vi "CASO.vi"() -> ()   [LabVIEW 2019]
uses:
  <vilib>/ActorFramework/Stop Msg/Stop Msg.lvclass
panel:
  in  "COMPRAR MERCANCÍA":bool
  in  "10 PESOS MEXICANOS":bool
  in  "5 PESOS MEXICANOS":bool
  in  "2 PESOS MEXICANOS":bool
  in  "1 PESO MEXICANO":bool
  in  "SOLICITAR MERCANCIA":bool
  out "PRECIO":dbl
  out "CANTIDAD":dbl
  out "PRODUCTO":string
  out "MONEDA":string
  in  "MERCANCÍA":i32(listbox)
  out "CRÉDITO":dbl
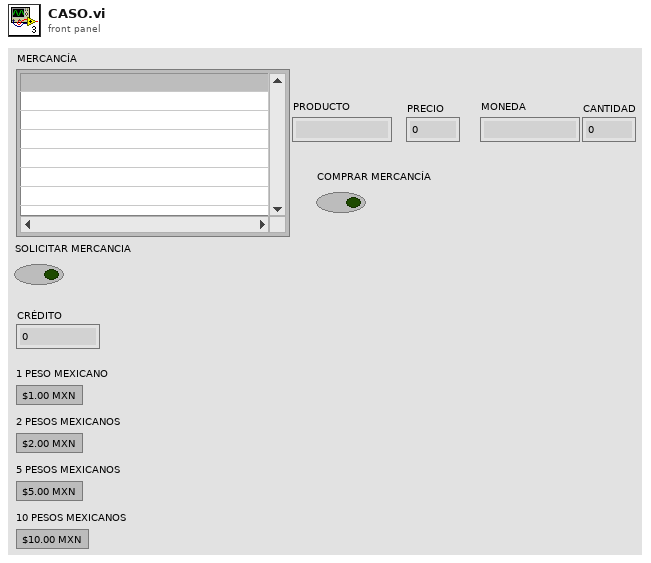
[diagram p1: front panel]
types:
  T1 = cluster{"CANTIDAD":dbl, "MONEDA":string, "PRECIO ":dbl, "PRODUCTO":string}
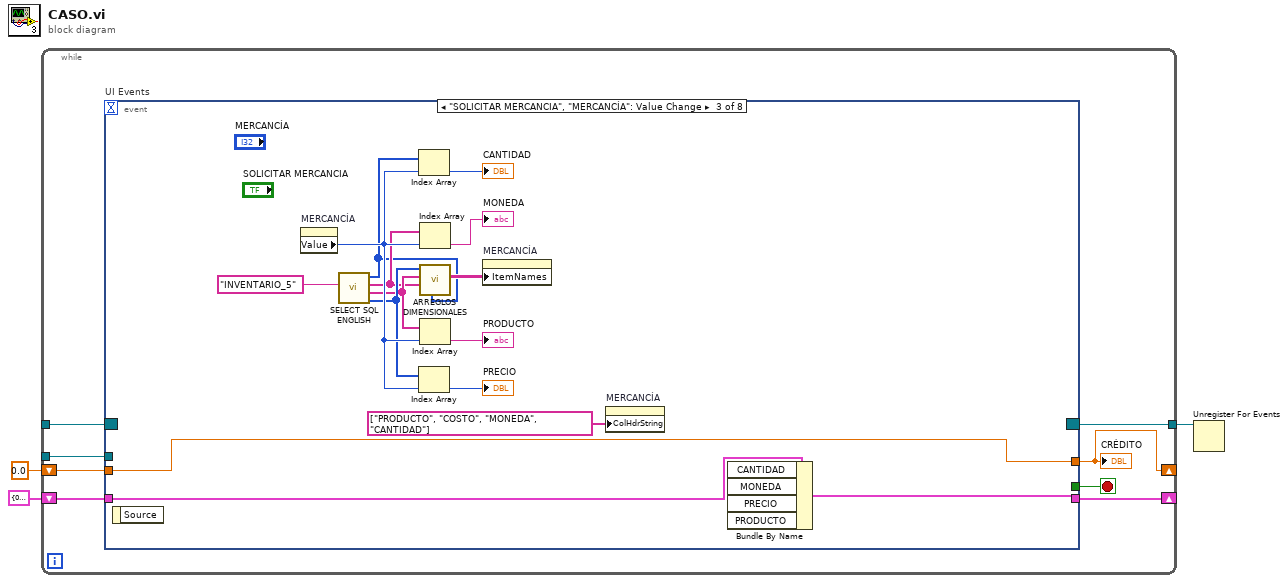
[diagram p0: block diagram]
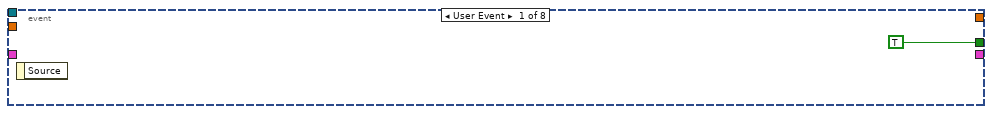
[diagram p2: hidden frame]
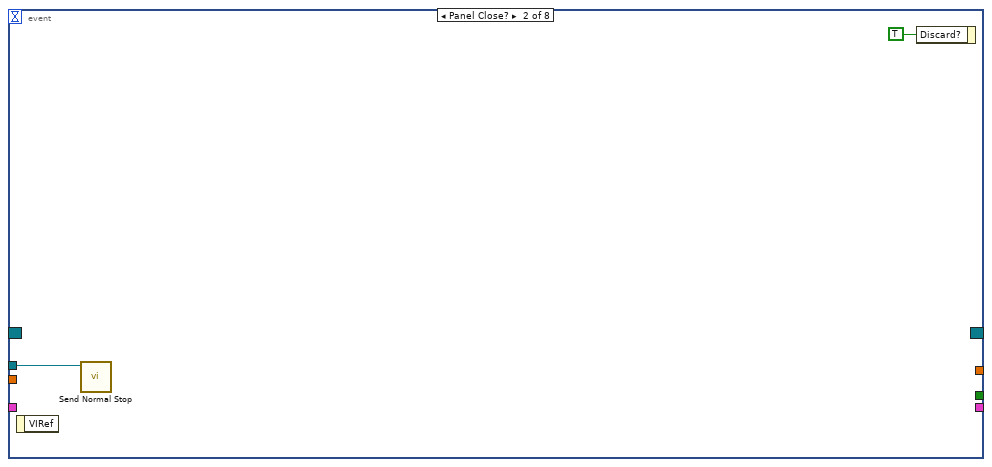
[diagram p3: hidden frame]
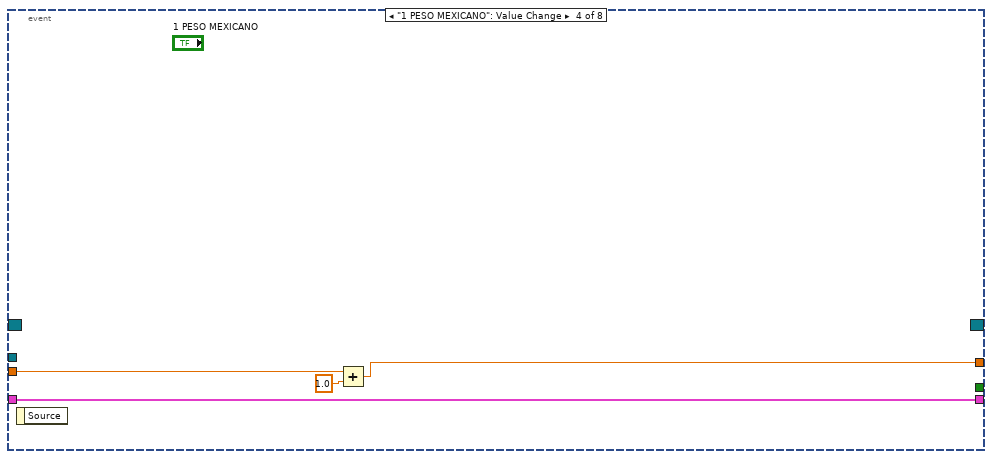
[diagram p4: hidden frame]
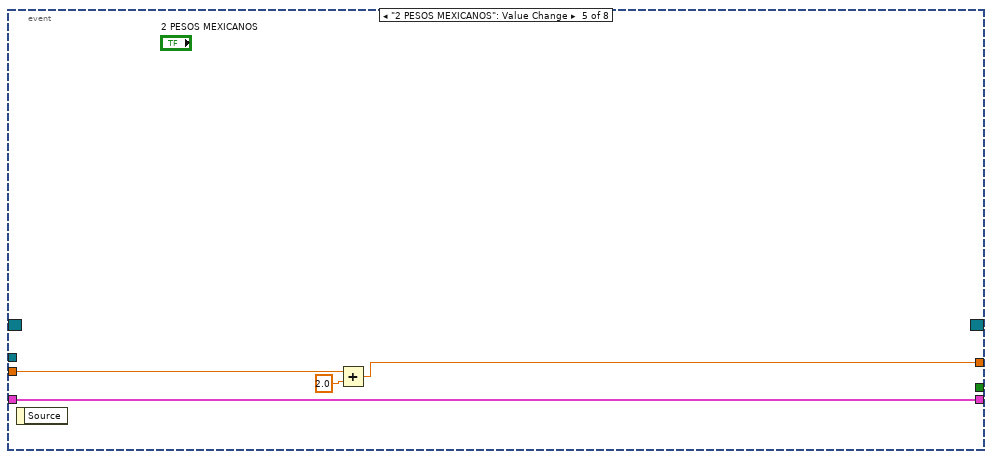
[diagram p5: hidden frame]
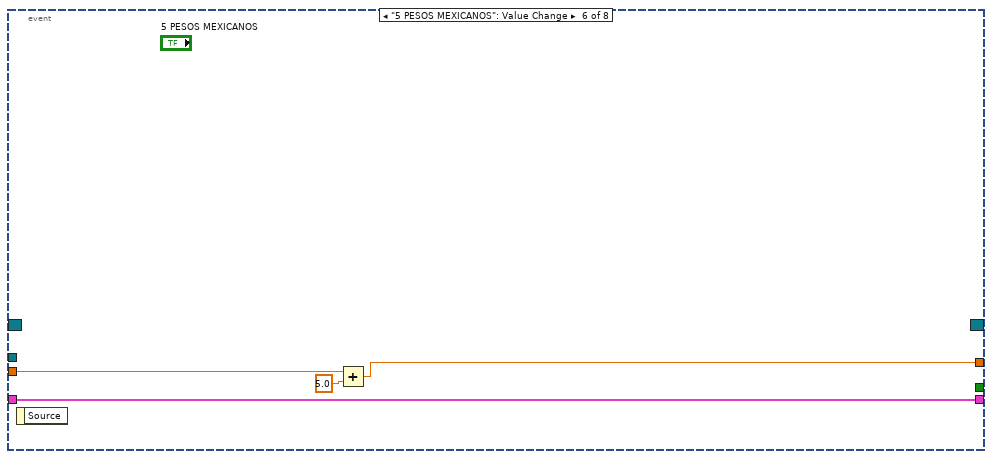
[diagram p6: hidden frame]
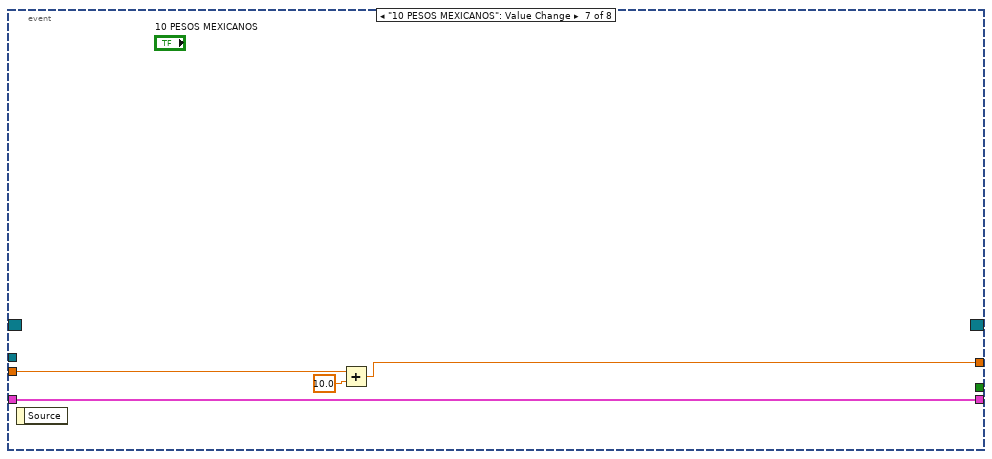
[diagram p7: hidden frame]
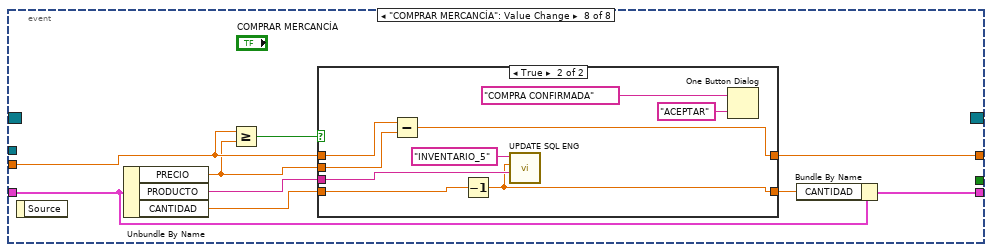
[diagram p8: hidden frame]
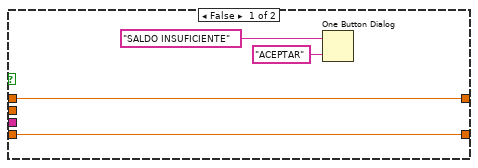
[diagram p9: hidden frame]
diagram:
  n1 = while {
    tunnel: [w12] -> w2
    tunnel: [w10] -> w1
    tunnel: _ -> [w9]
    shift-right: [w7] -> _
    shift-left: T1 {"CANTIDAD"=0.0, "MONEDA"="", "PRECIO "=0.0, "PRODUCTO"=""} -> [w8]
    shift-right: [w5] -> _
    shift-left: 0.0 -> [w6]
    stop <- w11 stop-if-true
    n2 = event "UI Events" shown="[2] \"SOLICITAR MERCANCIA\", \"MERCANCÍA\": Value Change" {
      selector: w12 -> [_ _ _ _ _ _ _ _]
      dyn-events: [_ _ _ _ _ _ _ _] -> w10
      timeout: _ -> [_ _ _ _ _ _ _ _]
      tunnel: [TRUE _ _ _ _ _ _ _] -> w11
      tunnel: w9 -> [_ w14 _ _ _ _ _ _]
      tunnel: w8 -> [_ _ w28 w34 w38 w42 w46 w55]
      tunnel: [_ _ w27 w34 w38 w42 w46 w51] -> w7
      tunnel: [_ _ w25 w31 w35 w39 w43 w47] -> w5
      tunnel: w6 -> [_ _ w25 w33 w37 w41 w45 w49]
      event User Event {
        n3 = event-data() -> ()  [unwired: 1 in, 1 out]
      }
      event Panel Close? {
        n4 = event-data() -> ()  [unwired: 1 in, 1 out]
        n5 = call <vilib>:"Send Normal Stop.vi"("Message Enqueuer"=w14) -> ()  [unwired: 10 in, 1 out]
        n6 = event-data("Discard?"=TRUE) -> ()  [unwired: 1 in, 1 out]
      }
      event "SOLICITAR MERCANCIA", "MERCANCÍA": Value Change {
        n7 = event-data() -> ()  [unwired: 1 in, 1 out]
        n8 = property on="MERCANCÍA" class="MCListbox (strict)"() -> ("Value"=w26:i32)  [unwired: 2 in, 2 out]
        n9 = call "SELECT SQL ENGLISH.vi"("INVENTARIO"="INVENTARIO_5") -> ("COSTO"=w19:i64[], "PRODUCTO"=w18:string[], "MONEDA"=w17:string[], "CANTIDAD"=w16:i64[])  [unwired: 7 in]
        n10 = Index Array(array=w16, index=w26) -> (element=→"CANTIDAD":i64)
        n11 = Index Array(array=w19, index=w26) -> (element=→"PRECIO":i64)
        n12 = Index Array(array=w17, index=w26) -> (element=→"MONEDA":string)
        n13 = call "ARREGLOS DIMENSIONALES.vi"("CANTIDAD"=w16, "MONEDA"=w17, "PRODUCTO"=w18, "COSTO"=w19) -> ("Array"=w29:string[][])  [unwired: 7 in]
        n14 = Index Array(array=w18, index=w26) -> (element=→"PRODUCTO":string)
        n15 = property on="MERCANCÍA" class="MCListbox (strict)"("ItemNames"=w29) -> ()  [unwired: 2 in, 2 out]
        n16 = property on="MERCANCÍA" class="MCListbox (strict)"("ColHdrString"=string[] ["PRODUCTO", "COSTO", "MONEDA", "CANTIDAD"] ("Column Header Strings[]")) -> ()  [unwired: 2 in, 2 out]
        n17 = Bundle By Name(cluster=w28) -> (w27:T1)  [unwired: 4 in]
      }
      event "1 PESO MEXICANO": Value Change {
        n18 = event-data() -> ()  [unwired: 1 in, 1 out]
        n19 = Add(x=w33, y=1.0) -> (x+y=w31:dbl)
      }
      event "2 PESOS MEXICANOS": Value Change {
        n20 = event-data() -> ()  [unwired: 1 in, 1 out]
        n21 = Add(x=w37, y=2.0) -> (x+y=w35:dbl)
      }
      event "5 PESOS MEXICANOS": Value Change {
        n22 = event-data() -> ()  [unwired: 1 in, 1 out]
        n23 = Add(x=w41, y=5.0) -> (x+y=w39:dbl)
      }
      event "10 PESOS MEXICANOS": Value Change {
        n24 = event-data() -> ()  [unwired: 1 in, 1 out]
        n25 = Add(x=w45, y=10.0) -> (x+y=w43:dbl)
      }
      event "COMPRAR MERCANCÍA": Value Change {
        n26 = event-data() -> ()  [unwired: 1 in, 1 out]
        n27 = Unbundle By Name(w55) -> ("PRECIO"=w48:dbl, "PRODUCTO"=w52:string, "CANTIDAD"=w53:dbl)
        n28 = Greater Or Equal?(x=w49, y=w48) -> (x >= y?=w54:bool)
        n29 = case shown="True" w54 {
          tunnel: w53 -> [w58 w66]
          tunnel: w52 -> [_ w61]
          tunnel: [w58 w60] -> w50
          tunnel: w49 -> [w59 w65]
          tunnel: w48 -> [_ w64]
          tunnel: [w59 w63] -> w47
          frame False {
            n30 = One Button Dialog(message="SALDO INSUFICIENTE", button name ("OK")="ACEPTAR") -> ()  [unwired: 1 out]
          }
          frame True {
            n31 = Subtract(x=w65, y=w64) -> (x-y=w63:dbl)
            n32 = Decrement(x=w66) -> (x-1=w60:dbl)
            n33 = call "UPDATE SQL ENG.vi"("PRODUCTO"=w61, "number"=w60, "TABLA"="INVENTARIO_5") -> ()  [unwired: 9 in]
            n34 = One Button Dialog(message="COMPRA CONFIRMADA", button name ("OK")="ACEPTAR") -> ()  [unwired: 1 out]
          }
        }
        n35 = Bundle By Name(cluster=w55, "CANTIDAD"=w50) -> (w51:T1)
      }
    }
    "CRÉDITO" <- w5
  }
  n36 = Unregister For Events(event registration refnum=w1) -> ()  [unwired: 1 in, 1 out]
